vi "Radians per Second to RPM (Vector).vi"(3 "radians per second":dbl[](array[numeric])) -> (1 "rpm":dbl[](array[numeric]))   [LabVIEW 2017, in "NI_Robotics Utilities.lvlib"]
doc: "Converts a 1D array of angular velocities from radians per second to rpm."
uses:
  <vilib>/robotics/Utilities/NI_Robotics Utilities.lvlib
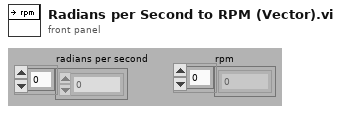
[diagram p1: front panel]
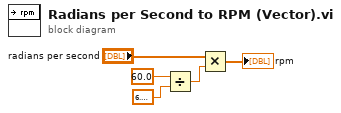
[diagram p0: block diagram]
diagram:
  n1 = Divide(x=60.0, y=6.283185307179586) -> (x/y=w5:dbl)
  n2 = Multiply(x="radians per second", y=w5) -> (x*y=→"rpm":dbl[])
